vi "OKNModelLog.vi"() -> ()   [LabVIEW 2016]
uses:
  Cerebellum/Cerebellum.lvclass
panel:
  out "rslip":dbl(graph)
  in  "Stim OFF?":bool
  out "Cereb":T1(graph)
  out "EyeVelocities":T2(graph)
  in  "Training":bool=TRUE
  out "SimPars":T3
  in  "stop":bool
  out "Log File name":string="DataLog__27Feb15p55"
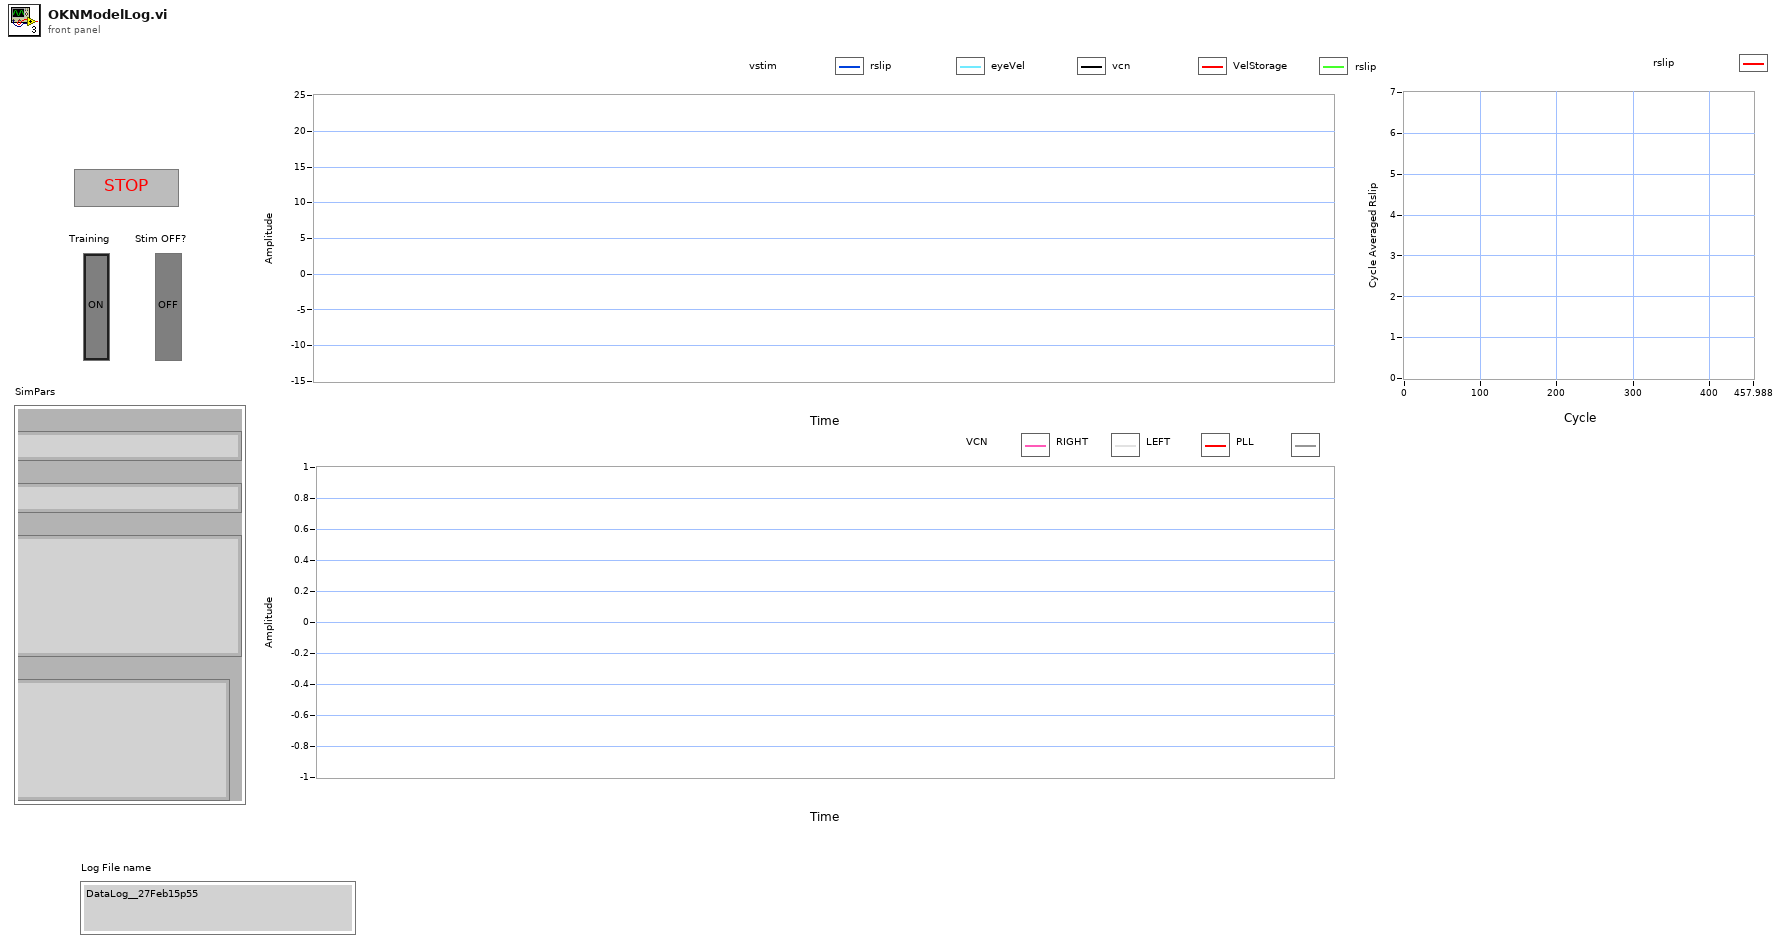
[diagram p1: front panel]
types:
  T1 = cluster{dbl, "PC Right":dbl, dbl, dbl, "Negwave":dbl}
  T2 = cluster{"eyeVel":dbl, dbl, "eyeVel":dbl, dbl, "Eye position":dbl}
  T3 = cluster{"RightNetwork":path, "LeftNetwork":path, "previewRight":string, "previewLeft":string}
  T4 = cluster{dbl, "PC Right":dbl, dbl, dbl, "Negwave":dbl}[]
  T5 = cluster{"eyeVel":dbl, dbl, "eyeVel":dbl, dbl, "Eye position":dbl}[]
  T6 = cluster{"square":dbl[], "3armonics":dbl[], "2armonics":dbl[], "1armonic":dbl[]}
  T7 = cluster{dbl, dbl, "eyeVel":dbl, dbl, "Eye position":dbl}
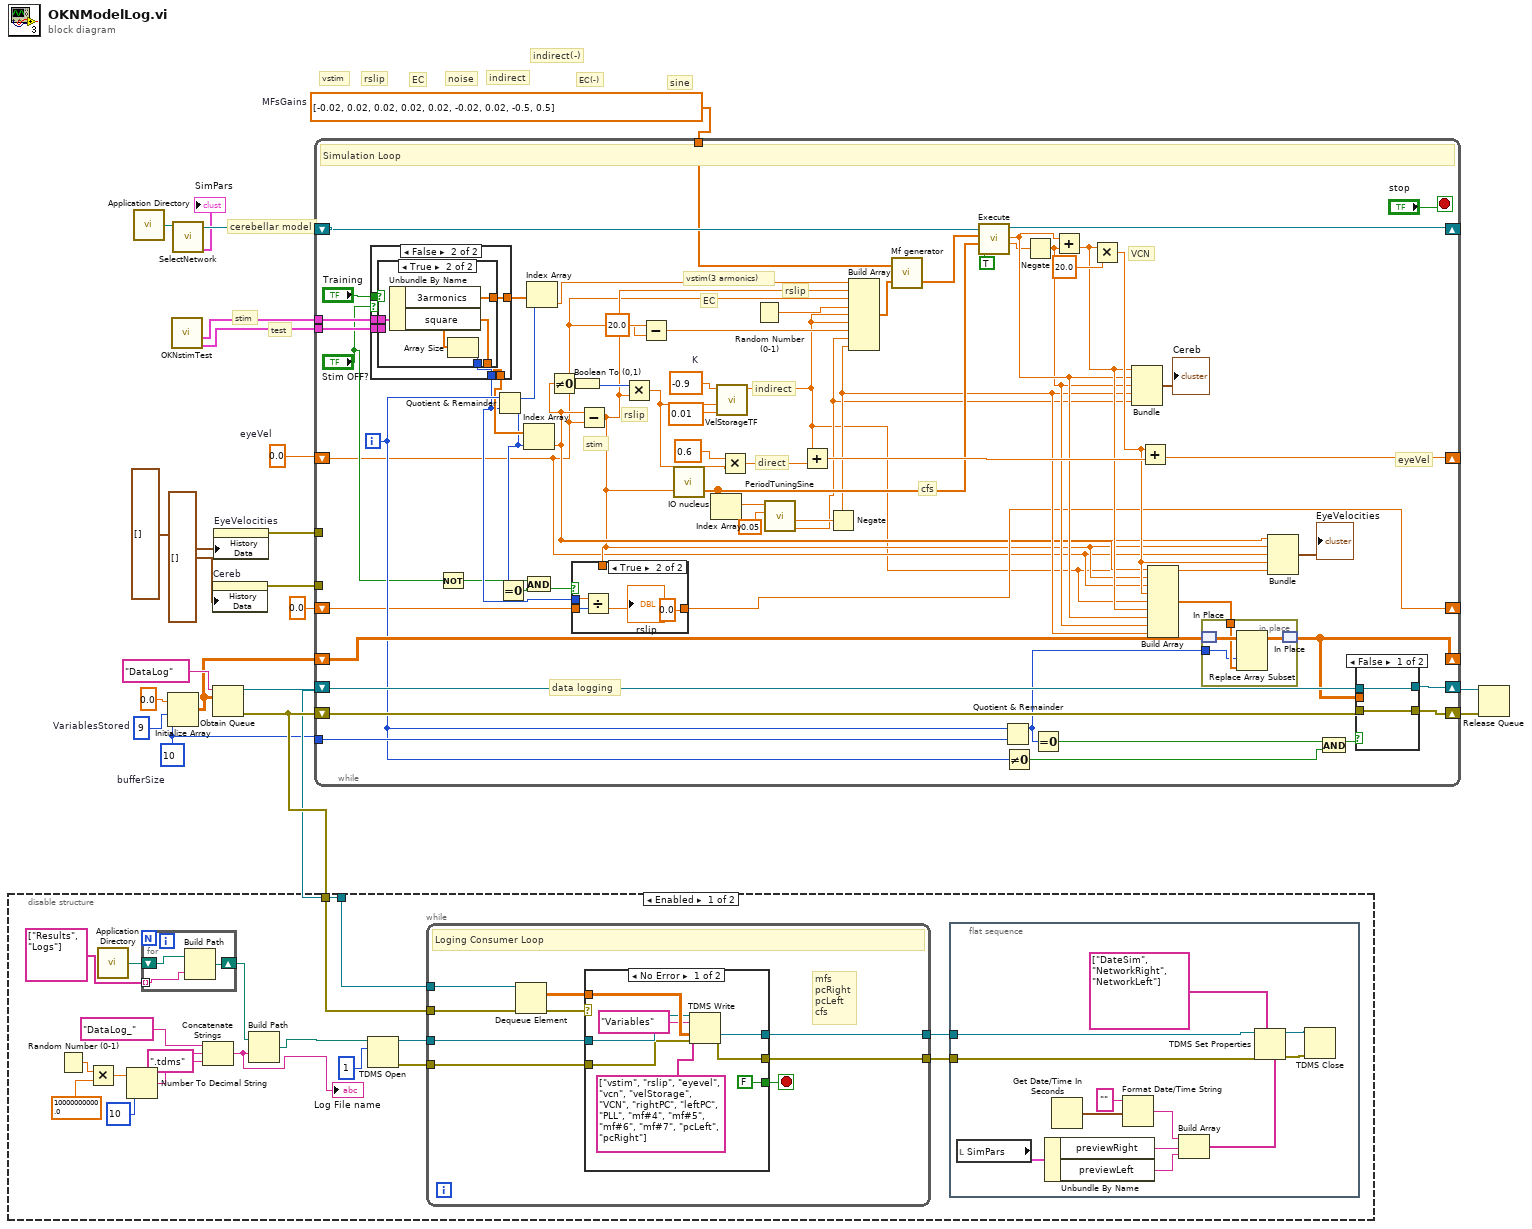
[diagram p0: block diagram]
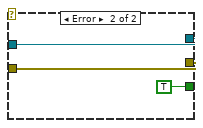
[diagram p2: hidden frame]
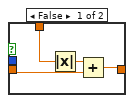
[diagram p4: hidden frame]
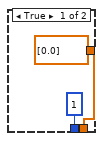
[diagram p5: hidden frame]
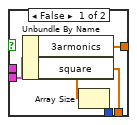
[diagram p6: hidden frame]
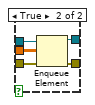
[diagram p7: hidden frame]
diagram:
  w6 = dbl[] [-0.02, 0.02, 0.02, 0.02, 0.02, -0.02, 0.02, -0.5, 0.5]  # MFsGains
  w9 = 0.0  # eyeVel
  w14 = 10  # bufferSize
  w18 = 9  # VariablesStored
  # "indirect(-)"
  # "EC(-)"
  # "indirect"
  # "noise"
  # "EC"
  # "sine"
  # "rslip"
  # "vstim"
  # "test"
  # "stim"
  # "cerebellar model"
  n1 = call <vilib>:"Application Directory.vi"() -> ("Application Directory"=w21:path)
  n2 = Initialize Array(0.0 ("element"), w18, w14) -> (w17:dbl[][])
  n3 = call "OKNstimTest.vi"() -> ("ComplexTest"=w7:T6, "ComplexStim"=w8:T6)  [unwired: 8 in, 2 out]
  n4 = call "SelectNetwork.vi"("base path"=w21) -> ("SimPars"=→"SimPars":T3, "Cerebellum out"=w11:refnum<class "Cerebellum.lvclass">)  [unwired: 9 in]
  n5 = property on="Cereb" class="WFChart (strict)"("History Data"=T4 []) -> (error out=w4:errorcluster)  [unwired: 2 in, 1 out]
  n6 = Obtain Queue(name (unnamed)="DataLog", element data type=w17) -> (queue out=w15:refnum<queue>, error out=w16:errorcluster)  [unwired: 3 in, 1 out]
  n7 = disable-structure shown="Enabled" {
    disable-tunnel: w15 -> [w40 _]
    disable-tunnel: w16 -> [w39 _]
    frame Enabled {
      n8 = Random Number (0-1)() -> (number: 0 to 1=w36:dbl)
      n9 = Multiply(x=w36, y=10000000000.0) -> (x*y=w34:dbl)
      n10 = call <vilib>:"Application Directory.vi"() -> ("Application Directory"=w30:path)
      n11 = Number To Decimal String(number=w34, width (-)=i16 10) -> (decimal integer string=w31:string)
      n12 = for {
        shift-right: [w55] -> w27
        shift-left: w30 -> [w54]
        tunnel: string[] ["Results", "Logs"] -> [w53] mode=indexing
        n13 = Build Path(base path=w54, name or relative path=w53) -> (appended path=w55:path)
      }
      n14 = Concatenate Strings("DataLog_" ("Header"), w31, ".tdms" ("string")) -> (w22:string)
      "Log File name" <- w22
      n15 = Build Path(base path=w27, name or relative path=w22) -> (appended path=w23:path)
      n16 = TDMS Open(10:i16 1 ("width (-)"), 11:w23) -> (0:w38:errorcluster, 3:w37:refnum<k34>)  [unwired: 5 in]
      n17 = while {
        tunnel: w37 -> [w62]
        tunnel: w38 -> [w58]
        tunnel: [w61] -> w26
        tunnel: [w60] -> w25
        tunnel: w40 -> [w57]
        tunnel: w39 -> [w59]
        stop <- w56 stop-if-true
        # "mfs\npcRight\npcLeft\ncfs"
        # "Loging Consumer Loop"
        n18 = Dequeue Element(queue=w57, error in (no error)=w59) -> (element=w63:dbl[][], error out=w64:errorcluster)  [unwired: 1 in, 2 out]
        n19 = case shown="No Error" w64 {
          tunnel: w63 -> [w72 _]
          tunnel: w62 -> [w71 w75]
          tunnel: w58 -> [w70 w74]
          tunnel: [w69 w75] -> w61
          tunnel: [w68 w74] -> w60
          tunnel: [FALSE TRUE] -> w56
          frame No Error {
            n20 = TDMS Write(0:w71, 5:"Variables" ("group name in (Untitled)"), 7:string[] ["vstim", "rslip", "eyevel", "vcn", "velStorage", "VCN", "rightPC", "leftPC", "PLL", "mf#4", "mf#5", "mf#6", "mf#7", "pcLeft", "pcRight"] ("channel name(s) in (Untitled)"), 9:w72, 11:w70) -> (4:w69:refnum<k34>, 15:w68:errorcluster)  [unwired: 1 in, 2 out]
          }
          frame Error {
          }
        }
      }
      n21 = flat-sequence {
        tunnel: w26 -> [w51]
        tunnel: w25 -> [w50]
        frame #0 {
          n22 = local read "SimPars"() -> (w47:T3)
          n23 = Unbundle By Name(w47) -> ("previewRight"=w46:string, "previewLeft"=w45:string)
          n24 = Get Date/Time In Seconds() -> (seconds since 1Jan1904=w44:timestamp)
          n25 = Format Date/Time String(time format string (%c)="", seconds (now)=w44) -> (date/time string=w43:string)  [unwired: 1 in]
          n26 = Build Array(w43, w46, w45) -> (w42:string[])
          n27 = TDMS Set Properties(5:w42, 7:string[] ["DateSim", "NetworkRight", "NetworkLeft"] ("property names"), 8:w50, 11:w51) -> (0:w48:errorcluster, 3:w49:refnum<k34>)  [unwired: 2 in, 2 out]
          n28 = TDMS Close(8:w48, 11:w49) -> ()  [unwired: 2 out]
        }
      }
    }
    frame Disabled {
    }
  }
  n29 = property on="EyeVelocities" class="WFChart (strict)"("History Data"=T5 []) -> (error out=w5:errorcluster)  [unwired: 2 in, 1 out]
  n30 = while {
    shift-right: [w117] -> _
    shift-left: w11 -> [w118]
    shift-right: [w139] -> w12
    shift-left: w15 -> [w138]
    shift-right: [w136] -> w13
    shift-left: w16 -> [w137]
    shift-right: [w130] -> _
    shift-left: w17 -> [w131]
    tunnel: w14 -> [w135]
    shift-right: [w109] -> _
    shift-left: w9 -> [w79]
    tunnel: w8 -> [w121]
    tunnel: w7 -> [w120]
    tunnel: w6 -> [w114]
    tunnel: w5 -> [_]
    tunnel: w4 -> [_]
    shift-right: [w92] -> _
    shift-left: 0.0 -> [w93]
    i -> [w122]
    stop <- "stop" stop-if-true
    w127 = -0.9  # K
    # "cfs"
    # "EC"
    # "rslip"
    # "vstim(3 armonics)"
    # "eyeVel"
    # "rslip"
    # "VCN"
    # "stim"
    # "direct"
    # "indirect"
    # "data logging"
    # "Simulation Loop"
    n31 = case shown="False" "Stim OFF?" {
      tunnel: "Training" -> [_ w155]
      tunnel: w121 -> [_ w154]
      tunnel: w120 -> [_ w153]
      tunnel: [w148 w152] -> w119
      tunnel: [1 w151] -> w91
      tunnel: [w148 w150] -> w103
      frame True {
        w148 = dbl[] [0.0] ("3armonics")
      }
      frame False {
        n32 = case shown="True" w155 {
          tunnel: w154 -> [_ w163]
          tunnel: w153 -> [w159 _]
          tunnel: [w158 w162] -> w152
          tunnel: [w157 w161] -> w151
          tunnel: [w156 w160] -> w150
          frame False {
            n33 = Unbundle By Name(w159) -> ("3armonics"=w158:dbl[], "square"=w156:dbl[])
            n34 = Array Size(array=w156) -> (size(s)=w157:i32)
          }
          frame True {
            n35 = Unbundle By Name(w163) -> ("3armonics"=w162:dbl[], "square"=w160:dbl[])
            n36 = Array Size(array=w160) -> (size(s)=w161:i32)
          }
        }
      }
    }
    n37 = Not(x="Stim OFF?") -> (.not. x?=w82:bool)
    n38 = Quotient & Remainder(x=w122, y=w91) -> (x-y*floor(x/y)=w95:i32)  [unwired: 1 out]
    n39 = Equal To 0?(x=w95) -> (x = 0?=w96:bool)
    n40 = Index Array(array=w103, index=w95) -> (element=w88:dbl)
    n41 = And(x=w82, y=w96) -> (x .and. y?=w84:bool)
    n42 = Index Array(array=w119, index=w95) -> (element=w89:dbl)
    n43 = Not Equal To 0?(x=w88) -> (x != 0?=w90:bool)
    n44 = Boolean To (0,1)(Boolean=w90) -> (0, 1=w86:i16)
    n45 = Subtract(x=w88, y=w79) -> (x-y=w80:dbl)
    n46 = case shown="True" w84 {
      tunnel: [w143 0.0] -> w92
      tunnel: w93 -> [w142 w147]
      tunnel: w80 -> [w141 _]
      tunnel: w91 -> [_ w146]
      frame False {
        n47 = Absolute Value(x=w141) -> (abs(x)=w140:dbl)
        n48 = Add(x=w140, y=w142) -> (x+y=w143:dbl)
      }
      frame True {
        n49 = Divide(x=w147, y=w146) -> (x/y=→"rslip":dbl)
      }
    }
    n50 = Multiply(x=w86, y=w80) -> (x*y=w85:dbl)
    n51 = Subtract(x=w79, y=20.0 ("x")) -> (x-y=w78:dbl)
    n52 = call "IO nucleus.vi"("cf"=w80) -> ("cfs"=w107:dbl[])  [unwired: 2 in]
    n53 = Index Array(array=w107) -> (element=w112:dbl)  [unwired: 1 in]
    n54 = call "VelStorageTF.vi"("Int. Step (ms)"=0.01, "Retinal Slip"=w85, "Leak cnt"=w127) -> ("Eye position"=w76:dbl)  [unwired: 8 in]
    n55 = Multiply(x=0.6, y=w85) -> (x*y=w123:dbl)
    n56 = Random Number (0-1)() -> (number: 0 to 1=w87:dbl)
    n57 = call "PeriodTuningSine.vi"("cfspont"=0.05, "cf_right"=w112) -> ("Negwave"=w97:dbl, "Postwave"=w110:dbl)  [unwired: 6 in, 2 out]
    n58 = Add(x=w76, y=w123) -> (x+y=w124:dbl)
    n59 = Negate(x=w110) -> (-x=w98:dbl)
    n60 = Build Array(w89, w80, w79, w87, w76, w76, w78, w97, w98) -> (w113:dbl[])
    n61 = call "Mf generator.vi"("Inputs"=w113, "Gains"=w114) -> ("Mfs Inputs"=w106:dbl[])  [unwired: 1 in]
    n62 = call "Execute.vi"("Active?"=TRUE, "cfs"=w107, "Inputs"=w106, "Cerebellum in"=w118) -> ("PC Left"=w81:dbl, "PC Right"=w100:dbl, "Cerebellum out"=w117:refnum<class "Cerebellum.lvclass">)  [unwired: 5 in]
    n63 = Quotient & Remainder(x=w122, y=w135) -> (x-y*floor(x/y)=w129:i32)  [unwired: 1 out]
    n64 = Not Equal To 0?(x=w122) -> (x != 0?=w132:bool)
    n65 = Negate(x=w81) -> (-x=w99:dbl)
    n66 = Equal To 0?(x=w129) -> (x = 0?=w134:bool)
    n67 = Add(x=w100, y=w99) -> (x+y=w101:dbl)
    n68 = Multiply(x=w101, y=20.0) -> (x*y=w102:dbl)
    n69 = Bundle(w101, "PC Right"=w100, w99, w98, "Negwave"=w97) -> (→"Cereb":T1)  [unwired: 1 in]
    n70 = Add(x=w102, y=w124) -> (x+y=w109:dbl)
    n71 = Build Array(w88, w80, w79, w102, w76, w101, w100, w99, w98) -> (w108:dbl[])
    n72 = in-place {
      in-place-border: w129 -> [w164]
      in-place-border: w108 -> [w165]
      n73 = in-place-match #1(w131) -> (w167:dbl[][])
      n74 = Replace Array Subset(array=w167, new element=w165, index (col)=w164) -> (w166:dbl[][])  [unwired: 1 in]
      n75 = in-place-match #1(w166) -> (w130:dbl[][])
    }
    n76 = Bundle(w88, w80, "eyeVel"=w79, w102, "Eye position"=w76) -> (→"EyeVelocities":T7)  [unwired: 1 in]
    n77 = And(x=w134, y=w132) -> (x .and. y?=w133:bool)
    n78 = case shown="False" w133 {
      tunnel: [w169 w174] -> w139
      tunnel: [w168 w173] -> w136
      tunnel: w138 -> [w169 w172]
      tunnel: w137 -> [w168 w171]
      tunnel: w130 -> [_ w170]
      frame False {
      }
      frame True {
        n79 = Enqueue Element(queue=w172, element=w170, error in (no error)=w171) -> (queue out=w174:refnum<queue>, error out=w173:errorcluster)  [unwired: 1 in, 1 out]
      }
    }
  }
  n80 = Release Queue(queue=w12, error in (no error)=w13) -> ()  [unwired: 1 in, 3 out]
